vi "Do.vi"(8 "error in (no error)":errorcluster, 10 "Actor in":refnum<class "Actor.lvclass">, 11 "Compl Notif with Error Msg":refnum<class "Compl Notif with Error Msg.lvclass">) -> (0 "error out":errorcluster, 2 "Actor out":refnum<class "Actor.lvclass">)   [LabVIEW 2023, in "Async Methods Actor.lvlib" / "Compl Notif with Error Msg.lvclass"]
doc: "This VI delivers the message to the actor by calling the appropriate method(s) on the actor."
uses:
  Compl Notif with Error Msg.lvclass
  C:/Projects/Async Methods Actor/Async Methods Actor/Async Methods Actor Messages/Completion Notification Msg/Completion Notification Msg.lvclass
  <vilib>/ActorFramework/Actor/Actor.lvclass
  Async Methods Actor/Async Methods Actor.lvclass
  Completion Notification Msg/Completion Notification Msg.lvclass/Completion Notification Msg.ctl
  Completion Notification Msg/Read Async Method Error.vi
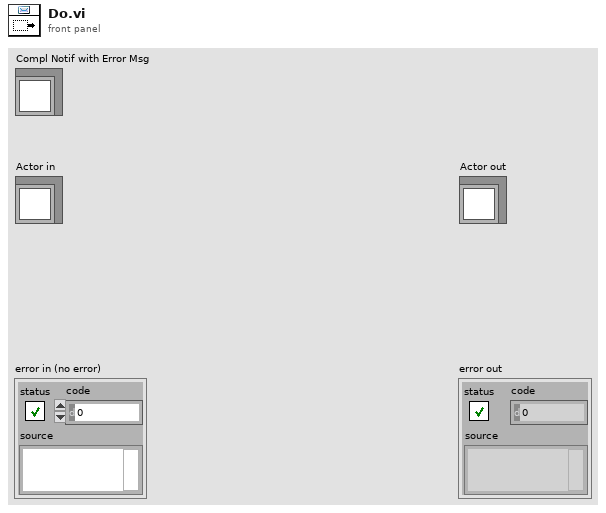
[diagram p1: front panel]
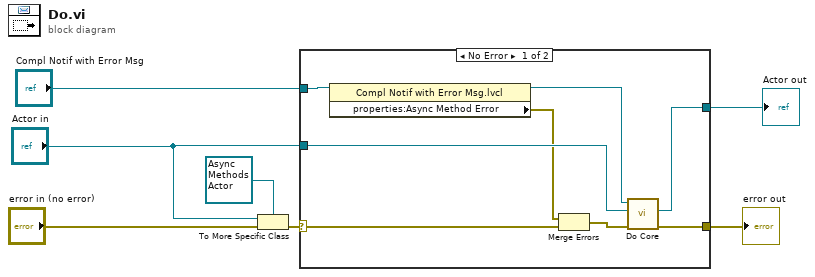
[diagram p0: block diagram]
diagram:
  n1 = To More Specific Class(target class=refnum<class "Async Methods Actor.lvclass"> refnum ("Actor in"), reference="Actor in", error in="error in (no error)") -> (error out=w6:errorcluster)  [unwired: 1 out]
  n2 = case shown="No Error" w6 {
    selector: w6 -> [w15 w17]
    tunnel: [w12 w17] -> w5
    tunnel: [w13 w16] -> w4
    tunnel: "Actor in" -> [w14 w16]
    tunnel: "Compl Notif with Error Msg" -> [w11 _]
    frame No Error {
      n3 = property class="Compl Notif with Error Msg.lvcl"(reference=w11) -> (reference out=w10:refnum<class "Compl Notif with Error Msg.lvclass">, "properties:Async Method Error"=w8:errorcluster)  [unwired: 1 in, 1 out]
      n4 = Merge Errors(w8, w15) -> (w9:errorcluster)
      n5 = call-dynamic "Do Core.vi"("error in (no error)"=w9, "Actor in"=w14, "Compl Notif with Error Msg"=w10) -> ("error out"=w12:errorcluster, "Actor out"=w13:refnum<class "Actor.lvclass">)  [unwired: 7 in]
    }
    frame Error {
      # "If type check fails, pass the original object out again."
    }
  }
  "error out" <- w5
  "Actor out" <- w4
